vi "subGetTargetFileName.vi"(11 "Refnum in":refnum<k20>) -> (3 "node text":string)   [LabVIEW 2020, in "SolutionBuilder.lvlib"]
uses:
  SolutionBuilder.lvlib
  <vilib>/xml/NI_XML.lvlib
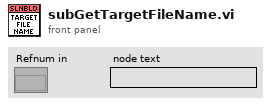
[diagram p1: front panel]
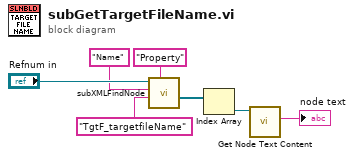
[diagram p0: block diagram]
diagram:
  n1 = call "subXMLFindNode.vi"("Node name"="Property", "Property value"="TgtF_targetfileName", "Property name"="Name", "Refnum in"="Refnum in") -> ("Nodes"=w5:refnum<k20>[])  [unwired: 6 in, 1 out]
  n2 = Index Array(array=w5) -> (element=w6:refnum<k20>)  [unwired: 1 in]
  n3 = call <vilib>:"Get Node Text Content.vi"("node in"=w6) -> ("node text"=→"node text":string)  [unwired: 8 in, 2 out]
